vi "SP_SetZTheta.vi"(6 "Theta Speed (10-100%)":dbl, 7 "Z Speed (10-100%)":dbl, 8 "error in (no error)":errorcluster, 9 "Theta in mdeg":dbl, 10 "Z in um":dbl, 11 "SemiProbe in":refnum<class "SemiProbe.lvclass">) -> (0 "error out":errorcluster, 3 "SemiProbe out":refnum<class "SemiProbe.lvclass">)   [LabVIEW 2018, in "SemiProbe.lvclass"]
uses:
  SemiProbe.lvclass
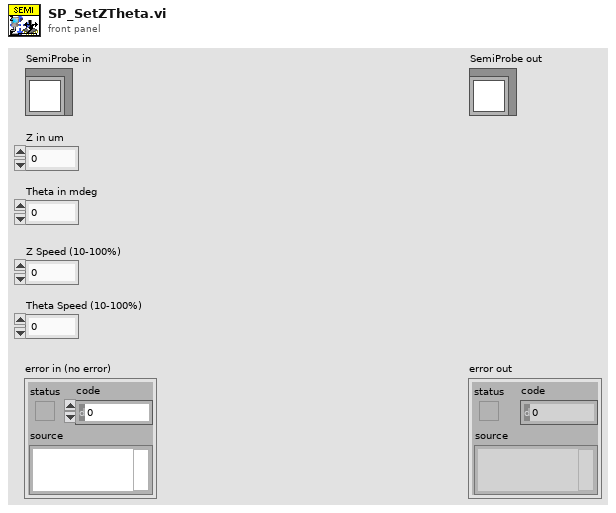
[diagram p1: front panel]
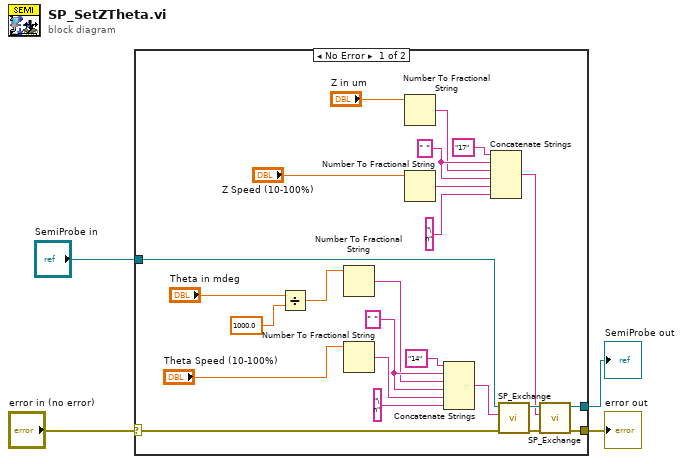
[diagram p0: block diagram]
diagram:
  n1 = case shown="No Error" "error in (no error)" {
    selector: "error in (no error)" -> [w22 w30]
    tunnel: [w11 w30] -> w3
    tunnel: [w12 w29] -> w1
    tunnel: "SemiProbe in" -> [w23 w29]
    frame No Error {
      w16 = " "
      w28 = " "
      n2 = Divide(x="Theta in mdeg", y=1000.0) -> (x/y=w5:dbl)
      n3 = Number To Fractional String(number=w5) -> (F-format string=w10:string)  [unwired: 3 in]
      n4 = Number To Fractional String(number="Theta Speed (10-100%)") -> (F-format string=w15:string)  [unwired: 3 in]
      n5 = Number To Fractional String(number="Z in um") -> (F-format string=w27:string)  [unwired: 3 in]
      n6 = Number To Fractional String(number="Z Speed (10-100%)") -> (F-format string=w20:string)  [unwired: 3 in]
      n7 = Concatenate Strings("14", w16, w10, w16, w15, "\n") -> (w9:string)
      n8 = Concatenate Strings("17", w28, w27, w28, w20, "\n") -> (w8:string)
      n9 = call-dynamic "SP_Exchange.vi"("error in (no error)"=w22, "command"=w9, "SemiProbe in"=w23) -> ("error out"=w14:errorcluster, "SemiProbe out"=w13:refnum<class "SemiProbe.lvclass">)  [unwired: 4 in, 3 out]
      n10 = call-dynamic "SP_Exchange.vi"("error in (no error)"=w14, "command"=w8, "SemiProbe in"=w13) -> ("error out"=w11:errorcluster, "SemiProbe out"=w12:refnum<class "SemiProbe.lvclass">)  [unwired: 4 in, 3 out]
    }
    frame Error {
    }
  }
  "error out" <- w3
  "SemiProbe out" <- w1
